vi "Read DAQ Params.vi"(11 "Template in":refnum<class "Template.lvclass">) -> (3 "DAQ Params":T1)   [LabVIEW 2020, in "Template.lvlib" / "Template.lvclass"]
uses:
  Template.lvclass
  typedefs/daq params.ctl
  Template.lvclass/Template.ctl
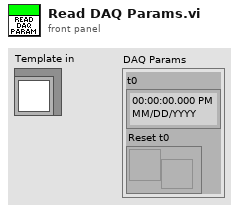
[diagram p1: front panel]
types:
  T1 = typedef "Template.lvlib/Template.lvclass/daq params.ctl" = cluster{"t0":timestamp, "Reset t0":refnum<notifier>}
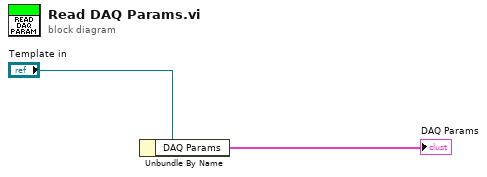
[diagram p0: block diagram]
diagram:
  n1 = Unbundle By Name("Template in") -> ("DAQ Params"=→"DAQ Params":T1)
